vi "GetCOMName.vi"(8 "Error In":errorcluster, 10 "COM Port":u32=1 min=1 step=1, 11 "VISA Resource List":string[](array[string])) -> (0 "Error Out":errorcluster, 2 "Found?":bool, 3 "VISA COM Resource Name":string)   [LabVIEW 2012, in "LV-Utilities.lvlib"]
uses:
  LV-Utilities.lvlib
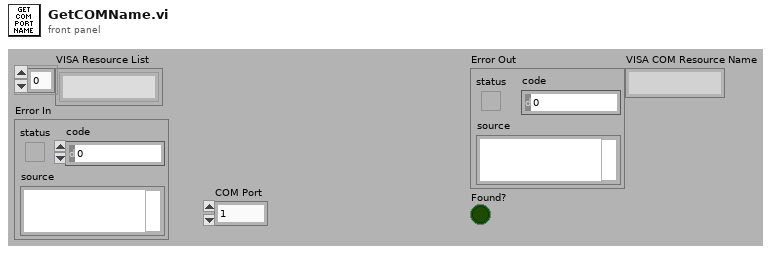
[diagram p1: front panel]
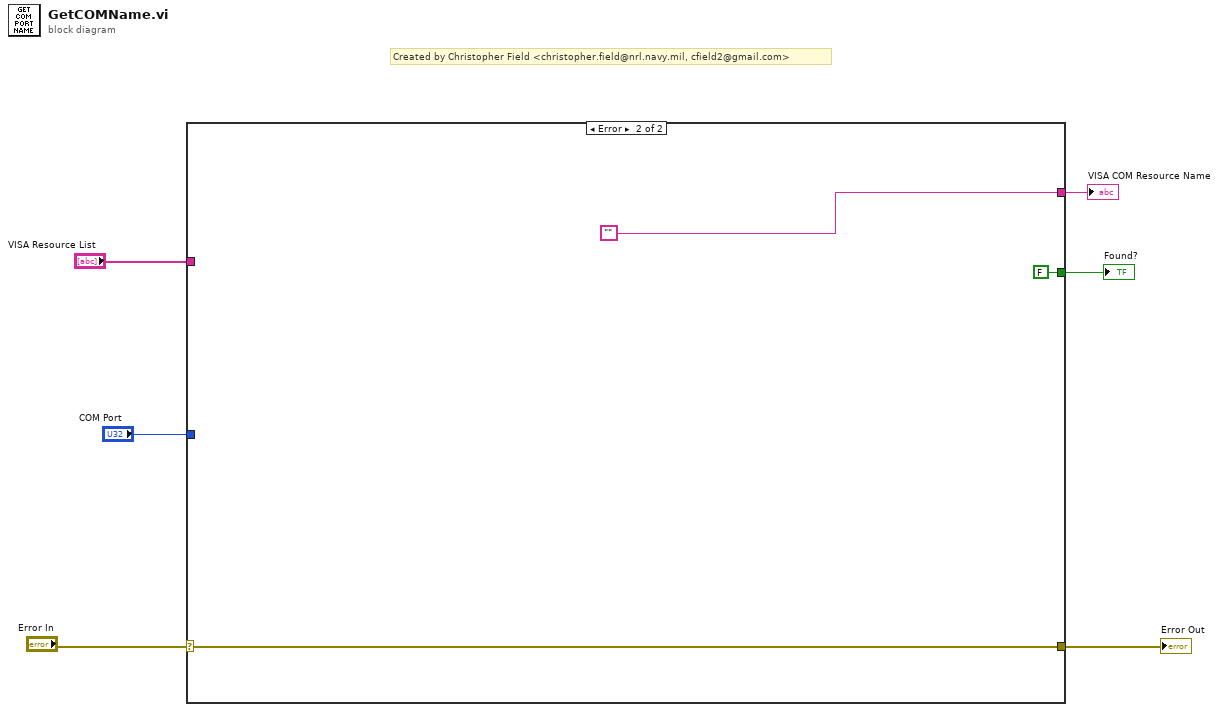
[diagram p0: block diagram]
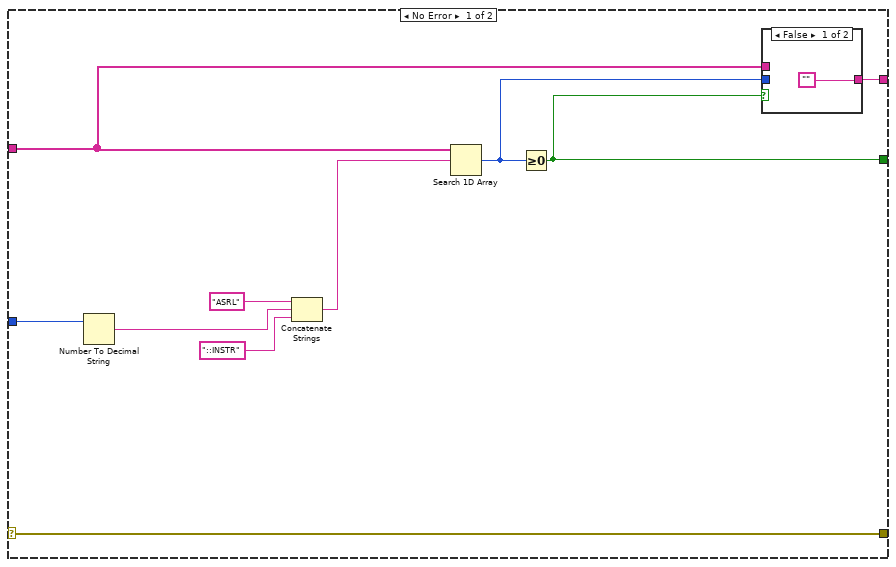
[diagram p2: hidden frame]
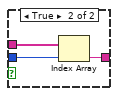
[diagram p3: hidden frame]
diagram:
  # "Created by Christopher Field <christopher.field@nrl.navy.mil, cfield2@gmail.com>"
  n1 = case shown="Error" "Error In" {
    selector: "Error In" -> [w15 w23]
    tunnel: "COM Port" -> [w16 _]
    tunnel: [w15 w23] -> w5
    tunnel: [w14 ""] -> w4
    tunnel: "VISA Resource List" -> [w10 _]
    tunnel: [w8 FALSE] -> w1
    frame No Error {
      n2 = Number To Decimal String(number=w16) -> (decimal integer string=w13:string)  [unwired: 1 in]
      n3 = Concatenate Strings("ASRL" ("regular expression"), w13, "::INSTR" ("regular expression")) -> (w9:string)
      n4 = Search 1D Array(1D array=w10, element=w9) -> (index of element=w7:i32)  [unwired: 1 in]
      n5 = Greater Or Equal To 0?(x=w7) -> (x >= 0?=w8:bool)
      n6 = case shown="False" w8 {
        tunnel: ["" w20] -> w14
        tunnel: w10 -> [_ w19]
        tunnel: w7 -> [_ w18]
        frame False {
        }
        frame True {
          n7 = Index Array(array=w19, index=w18) -> (element=w20:string)
        }
      }
    }
    frame Error {
    }
  }
  "Error Out" <- w5
  "VISA COM Resource Name" <- w4
  "Found?" <- w1
